vi "Cycle Average and RMS 1 chan (obs).vi"(6 "percent level settings":T2={"method"=enum."auto select", "histogram size"=256, "histogram method"=enum."mode", "reserved"=1.0} {"reserved" format="%0.2f"}, 7 "cycle number (1)":i32=1 min=1, 8 "error in (no error)":errorcluster, 9 "reference levels":T3={"high ref level"=90.0, "mid ref level"=50.0, "low ref level"=10.0, "ref units"=1} {"ref units" items=["absolute", "percent"]; "high ref level" format="%0.2f"; "low ref level" format="%0.2f"; "mid ref level" format="%0.2f"}, 11 "signal in":waveform(dbl)={"t0"=timestamp(0 s since 1904-01-01), "dt"=0.0, "Y"=[]}) -> (0 "error out":errorcluster, 2 "cycle RMS":dbl format="%.2g", 3 "cycle average":dbl format="%.2p", 4 "measurement info":T1 {"ref levels"."ref units" items=["absolute", "relative"]; "ref levels"."high ref level" format="%.2p"; "ref levels"."low ref level" format="%.2p"; "ref levels"."mid ref level" format="%.2p"; "end time" format="%.2p"; "start time" format="%.2p"})   [LabVIEW 2020, in "NI_MAPro.lvlib"]
uses:
  NI_MAPro.lvlib
  <resource>/lvanlys.dll
  NI_MABase.lvlib
panel:
  # "This VI is obsolete !!!\nYou should replace this VI in your diagram with the Cycle Average and RMS VI."
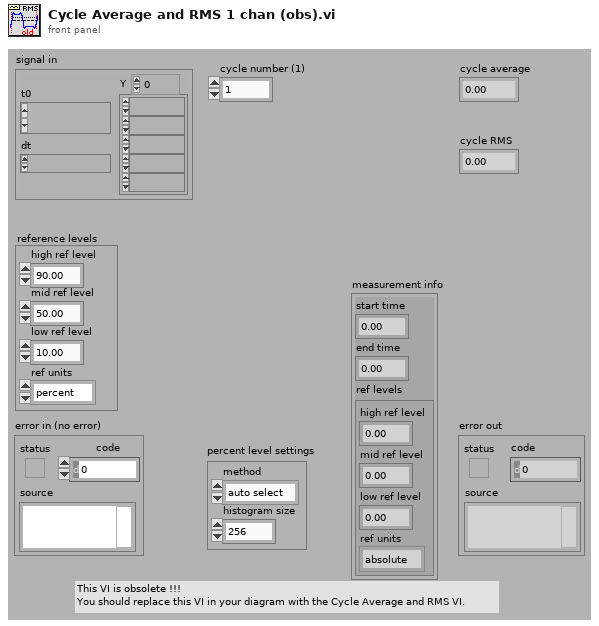
[diagram p1: front panel]
types:
  T1 = cluster{"start time":dbl, "end time":dbl, "ref levels":cluster{"high ref level":dbl, "mid ref level":dbl, "low ref level":dbl, "ref units":u16}}
  T2 = cluster{"method":enum32{"histogram", "peak", "auto select"}, "histogram size":i32, "histogram method":enum16{"mode"}, "reserved":dbl}
  T3 = cluster{"high ref level":dbl, "mid ref level":dbl, "low ref level":dbl, "ref units":u16}
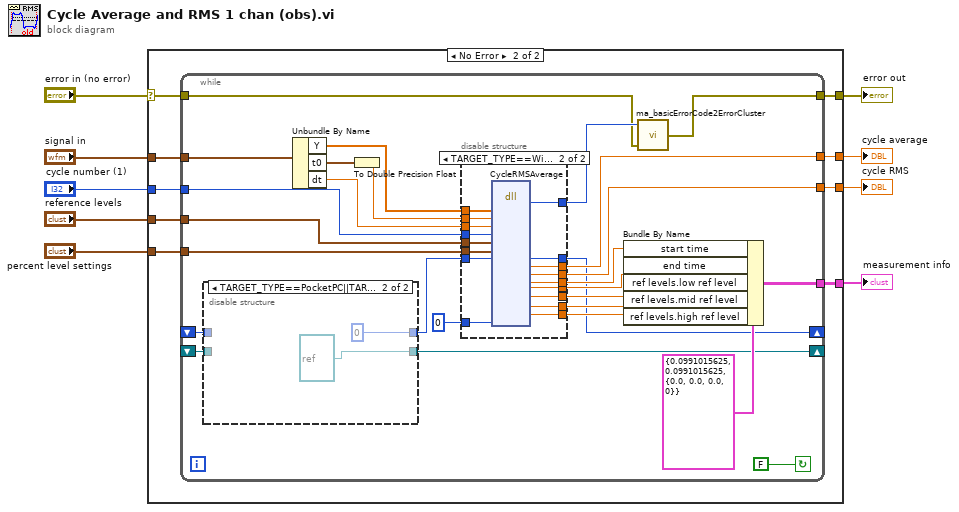
[diagram p0: block diagram]
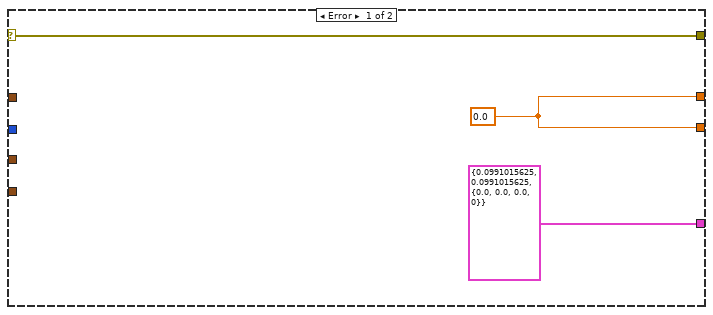
[diagram p2: hidden frame]
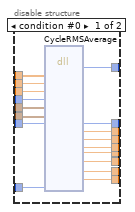
[diagram p3: hidden frame]
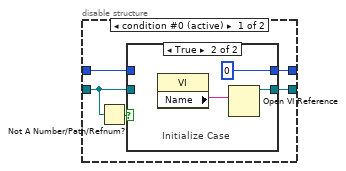
[diagram p4: hidden frame]
diagram:
  n1 = case shown="No Error" "error in (no error)" {
    selector: "error in (no error)" -> [w12 w20]
    tunnel: "reference levels" -> [_ w14]
    tunnel: "percent level settings" -> [_ w15]
    tunnel: "cycle number (1)" -> [_ w16]
    tunnel: "signal in" -> [_ w21]
    tunnel: [w12 w19] -> w4
    tunnel: [w11 w17] -> w3
    tunnel: [w11 w18] -> w2
    tunnel: [T1 {"start time"=0.0991015625, "end time"=0.0991015625, "ref levels"={"high ref level"=0.0, "mid ref level"=0.0, "low ref level"=0.0, "ref units"=0}} ("measurement info") w13] -> w1
    frame Error {
      w11 = 0.0 ("result")
    }
    frame No Error {
      n2 = while {
        tunnel: w21 -> [w48]
        tunnel: w20 -> [w23]
        tunnel: [w22] -> w19
        tunnel: [w32] -> w18
        tunnel: [w31] -> w17
        tunnel: w16 -> [w42]
        tunnel: w15 -> [w41]
        tunnel: w14 -> [w40]
        tunnel: [w39] -> w13
        shift-right: [w30] -> _
        shift-left: _ -> [w29]
        shift-right: [w26] -> _
        shift-left: _ -> [w28]
        stop <- FALSE continue-if-true
        n3 = disable-structure shown="TARGET_TYPE==PocketPC||TARGET_TYPE==PalmOS||TARGET_TYPE==FPGA||TARGET_TYPE==Embedded" {
          disable-tunnel: w28 -> [w85 _]
          disable-tunnel: [w86 refnum<vi> refnum ("VI Refnum")] -> w26
          disable-tunnel: w29 -> [w84 _]
          disable-tunnel: [w83 0 ("t")] -> w27
          frame condition #0 (active) {
            n4 = Not A Number/Path/Refnum?(number/path/refnum=w85) -> (NaN/Path/Refnum?=w87:bool)
            n5 = case shown="True" w87 {
              tunnel: [w89 w91] -> w86
              tunnel: w85 -> [w89 _]
              tunnel: w84 -> [w88 _]
              tunnel: [w88 0 ("error")] -> w83
              frame False {
              }
              frame True {
                # "Initialize Case"
                n6 = property class="VI"() -> ("Name"=w90:string)  [unwired: 2 in, 2 out]
                n7 = Open VI Reference(vi path=w90) -> (vi reference=w91:refnum<vi>)  [unwired: 1 in, 5 out]
              }
            }
          }
          frame condition #1 {
          }
        }
        n8 = Unbundle By Name(w48) -> ("Y"=w47:dbl[], "t0"=w45:timestamp, "dt"=w43:dbl)
        n9 = To Double Precision Float(number=w45) -> (double precision float=w44:dbl)
        n10 = disable-structure shown="TARGET_TYPE==Windows||TARGET_TYPE==Mac||TARGET_TYPE==Unix||TARGET_BITNESS==64" {
          disable-tunnel: w47 -> [w65 w82]
          disable-tunnel: [w64 w81] -> w24
          disable-tunnel: w44 -> [w63 w80]
          disable-tunnel: w43 -> [w62 w79]
          disable-tunnel: w42 -> [w61 w78]
          disable-tunnel: w41 -> [w60 w77]
          disable-tunnel: w40 -> [w59 w76]
          disable-tunnel: [w58 w75] -> w37
          disable-tunnel: [w57 w74] -> w36
          disable-tunnel: [w56 w73] -> w35
          disable-tunnel: [w55 w72] -> w34
          disable-tunnel: [w54 w71] -> w33
          disable-tunnel: [w53 w70] -> w32
          disable-tunnel: [w52 w69] -> w31
          disable-tunnel: [w51 w68] -> w30
          disable-tunnel: w27 -> [w50 w67]
          disable-tunnel: 0 ("newAlgorithm") -> [w49 w66]
          frame condition #0 {
            n11 = dll-call lib="C:/Program Files (x86)/National Instruments/LabVIEW 2020/resource/lvanlys.*" fn="CycleRMSAverage"("xH"=w65, "Xo"=w63, "dx"=w62, "cycleNum"=w61, "refLevel"=w59, "percentLevel"=w60, "work"=w50, "newAlgorithm"=w49) -> ("return type"=w64:i32, "work"=w51:i32, "cycleAvg"=w52:dbl, "cycleRMS"=w53:dbl, "startingTime"=w54:dbl, "endingTime"=w55:dbl, "lowRefLevel"=w56:dbl, "midRefLevel"=w57:dbl, "highRefLevel"=w58:dbl)  [unwired: 17 in, 2 out]
          }
          frame condition #1 (active) {
            n12 = dll-call lib="C:/Program Files (x86)/National Instruments/LabVIEW 2020/resource/lvanlys.dll" fn="CycleRMSAverage"("xH"=w82, "Xo"=w80, "dx"=w79, "cycleNum"=w78, "refLevel"=w76, "percentLevel"=w77, "work"=w67, "newAlgorithm"=w66) -> ("return type"=w81:i32, "work"=w68:i64, "cycleAvg"=w69:dbl, "cycleRMS"=w70:dbl, "startingTime"=w71:dbl, "endingTime"=w72:dbl, "lowRefLevel"=w73:dbl, "midRefLevel"=w74:dbl, "highRefLevel"=w75:dbl)  [unwired: 8 in, 11 out]
          }
        }
        n13 = Bundle By Name(cluster=T1 {"start time"=0.0991015625, "end time"=0.0991015625, "ref levels"={"high ref level"=0.0, "mid ref level"=0.0, "low ref level"=0.0, "ref units"=0}} ("measurement info"), "start time"=w33, "end time"=w34, "ref levels.low ref level"=w35, "ref levels.mid ref level"=w36, "ref levels.high ref level"=w37) -> (w39:T1)
        n14 = call "ma_basicErrorCode2ErrorCluster.vi"("error in (no error)"=w23, "Error Code"=w24) -> ("error out"=w22:errorcluster)  [unwired: 1 in]
      }
    }
  }
  "cycle average" <- w3
  "cycle RMS" <- w2
  "error out" <- w4
  "measurement info" <- w1
